vi "DB Select Data(count).vi"(7 "condition":string, 8 "error in (no error)":errorcluster, 10 "table":string, 11 "connection reference":T1) -> (0 "error out":errorcluster, 2 "Count":i32, 3 "connection reference out":T1)   [LabVIEW 2014]
uses:
  <vilib>/addons/database/NI_Database_API.lvlib
  <vilib>/addons/database/Connection.llb/Conn Execute.vi
  <vilib>/addons/database/Recordset.llb/Rec Fetch Recordset Data (R).vi
  <vilib>/addons/database/Recordset.llb/Rec Destroy - Connection.vi
  <vilib>/addons/database/_DB Variant To Data/Database Variant To Data.xnode
  <vilib>/addons/database/Connection.llb/Conn ObjectReference.ctl
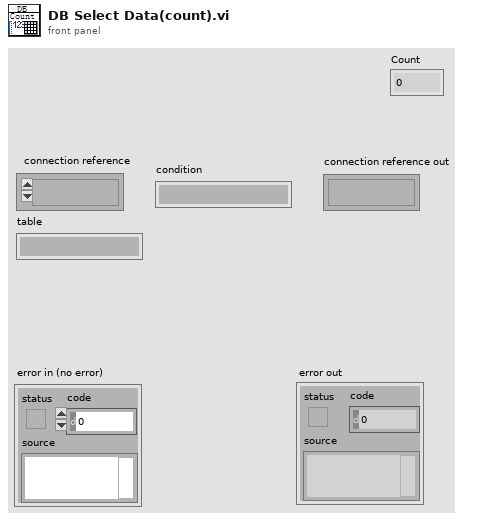
[diagram p1: front panel]
types:
  T1 = typedef "NI_Database_API.lvlib/Conn ObjectReference.ctl" = refnum<k1>
  T2 = typedef "NI_Database_API.lvlib/Rec ObjectReference.ctl" = refnum<k1>
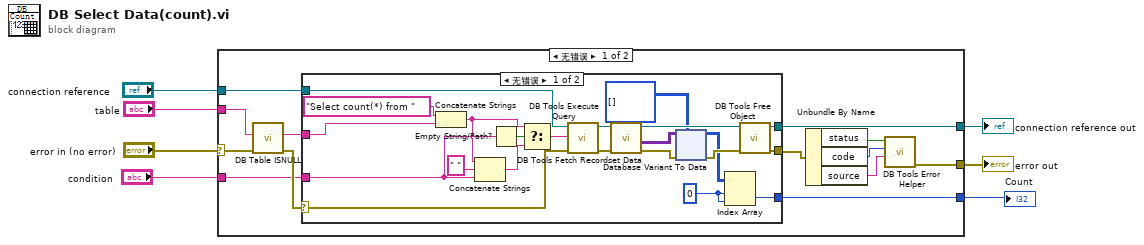
[diagram p0: block diagram]
diagram:
  n1 = case shown="无错误" "error in (no error)" {
    selector: "error in (no error)" -> [w9 w90]
    tunnel: "table" -> [w20 _]
    tunnel: [w13 w90] -> w6
    tunnel: [w12 w89] -> w5
    tunnel: "connection reference" -> [w11 w89]
    tunnel: "condition" -> [w10 _]
    tunnel: [w8 _] -> w1
    frame No Error {
      n2 = call "DB Table ISNULL.vi"("error in (no error)"=w9, "table"=w20) -> ("error out"=w17:errorcluster, "table out"=w18:string)  [unwired: 8 in]
      n3 = case shown="无错误" w17 {
        selector: w17 -> [w31 w88]
        tunnel: w18 -> [w29 _]
        tunnel: [w42 w88] -> w19
        tunnel: [w34 w87] -> w12
        tunnel: w11 -> [w32 w87]
        tunnel: w10 -> [w33 _]
        tunnel: [w21 _] -> w8
        frame No Error {
          w22 = 0 ("索引 (行)")
          n4 = Concatenate Strings("Select count(*) from ", w29) -> (w28:string)
          n5 = Concatenate Strings(w28, " " ("Substring"), w33) -> (w37:string)
          n6 = Empty String/Path?(string/path=w33) -> (empty?=w38:bool)
          n7 = Select(t=w28, s=w38, f=w37) -> (s? t:f=w35:string)
          n8 = call-poly <vilib>:"DB Tools Execute Query.vi"("error in (no error)"=w31, "SQL query"=w35, "connection reference"=w32) -> ("error out"=w39:errorcluster, "recordset reference"=w40:T2)  [unwired: 5 in]
          n9 = call-poly <vilib>:"DB Tools Fetch Recordset Data.vi"("error in (no error)"=w39, "recordset reference"=w40) -> ("error out"=w27:errorcluster, "recordset data"=w26:variant[][], "recordset reference out"=w41:T2)  [unwired: 3 in]
          n10 = xnode "Database Variant To Data"("database variant"=w26, "error in (no error)"=w27, "type"=i32[][] []) -> ("data"=w23:i32[][], "error out"=w24:errorcluster)
          n11 = Index Array(array=w23, index (row)=w22, index (col)=w22) -> (element=w21:i32)
          n12 = call-poly <vilib>:"DB Tools Free Object.vi"("error in (no error)"=w24, "recordset reference"=w41) -> ("error out"=w42:errorcluster, "connection reference"=w34:T1)  [unwired: 8 in]
        }
        frame Error {
        }
      }
      n13 = Unbundle By Name(w19) -> ("status"=w16:bool, "code"=w15:i32, "source"=w14:string)
      n14 = call <vilib>:"DB Tools Error Helper.vi"("source"=w14, "code"=w15, "status"=w16) -> ("error out"=w13:errorcluster)  [unwired: 8 in]
    }
    frame Error {
    }
  }
  "error out" <- w6
  "connection reference out" <- w5
  "Count" <- w1
